vi "Prep Status.vi"(8 "error in (no error)":errorcluster, 10 "Log":string, 11 "LogHTTPController in":refnum<class "LogHTTPController.lvclass">) -> (0 "error out":errorcluster, 2 "Response":refnum<class "Response.lvclass">, 3 "LogHTTPController out":refnum<class "LogHTTPController.lvclass">)   [LabVIEW 2020, in "VolatusData.lvlib" / "LogHTTPController.lvclass"]
uses:
  LogHTTPController.lvclass
  lv-http-util/HTTP Utils/Response/Response.lvclass
  Volatus/StringValue/StringValue.lvclass
  LogHTTPController.lvclass/LogHTTPController.ctl
  Volatus/MessageQ/MessageQ.lvclass
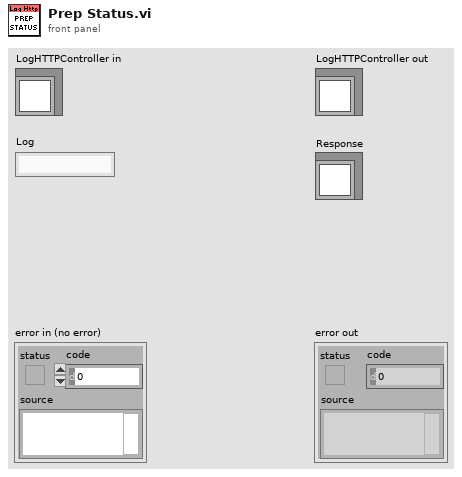
[diagram p1: front panel]
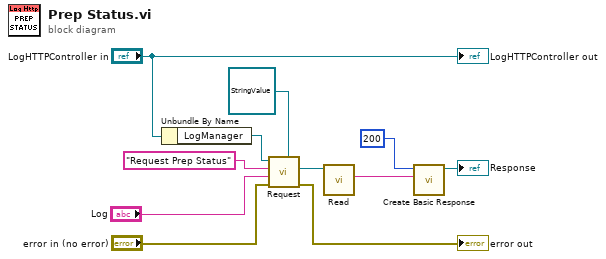
[diagram p0: block diagram]
diagram:
  n1 = Unbundle By Name("LogHTTPController in") -> ("LogManager"=w10:refnum<class "MessageQ.lvclass">)
  n2 = call "Request.vi"("Response Type (None)"=refnum<class "StringValue.lvclass"> refnum ("Volatus:StringValue.lvclass"), "error in (no error)"="error in (no error)", "Data"="Log", "ID"="Request Prep Status", "MessageQ in"=w10) -> ("error out"=→"error out":errorcluster, "Response"=w4:refnum<class "StringValue.lvclass">)  [unwired: 4 in, 1 out]
  n3 = call "Read.vi"("StringValue in"=w4) -> ("Value"=w3:string)  [unwired: 10 in]
  n4 = call "Create Basic Response.vi"("Payload"=w3, "Status Code"=u16 200) -> ("Response out"=→"Response":refnum<class "Response.lvclass">)  [unwired: 8 in, 1 out]
  "LogHTTPController out" <- "LogHTTPController in"
